vi "excel写.vi"(0 "路径":path, 1 "Table":string[][](table)=[["1", "2", "3", "4", "5", "6", "7", "8", "9", "10"], ["10", "11", "12", "13", "14", "15", "16", "17", "18", "19"], ["20", "21", "22", "23", "24", "25", "26", "27", "28", "29"], ["30", "31", "32", "33", "34", "35", "36", "37", "38", "39"]], 2 "数值":i8=1) -> ()   [LabVIEW 2011]
doc: "This VI demonstrates the use of ActiveX to write a table into a Microsoft Excel worksheet."
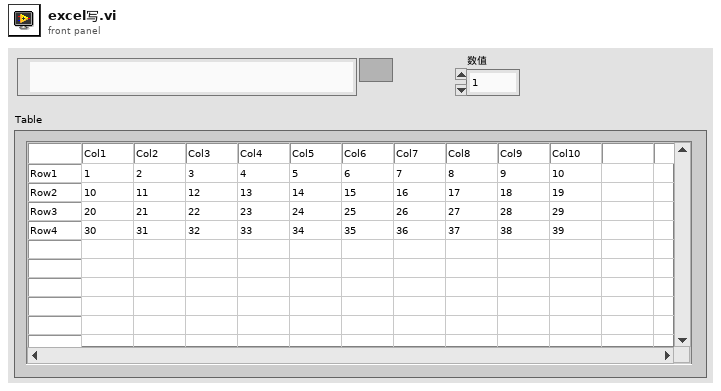
[diagram p1: front panel]
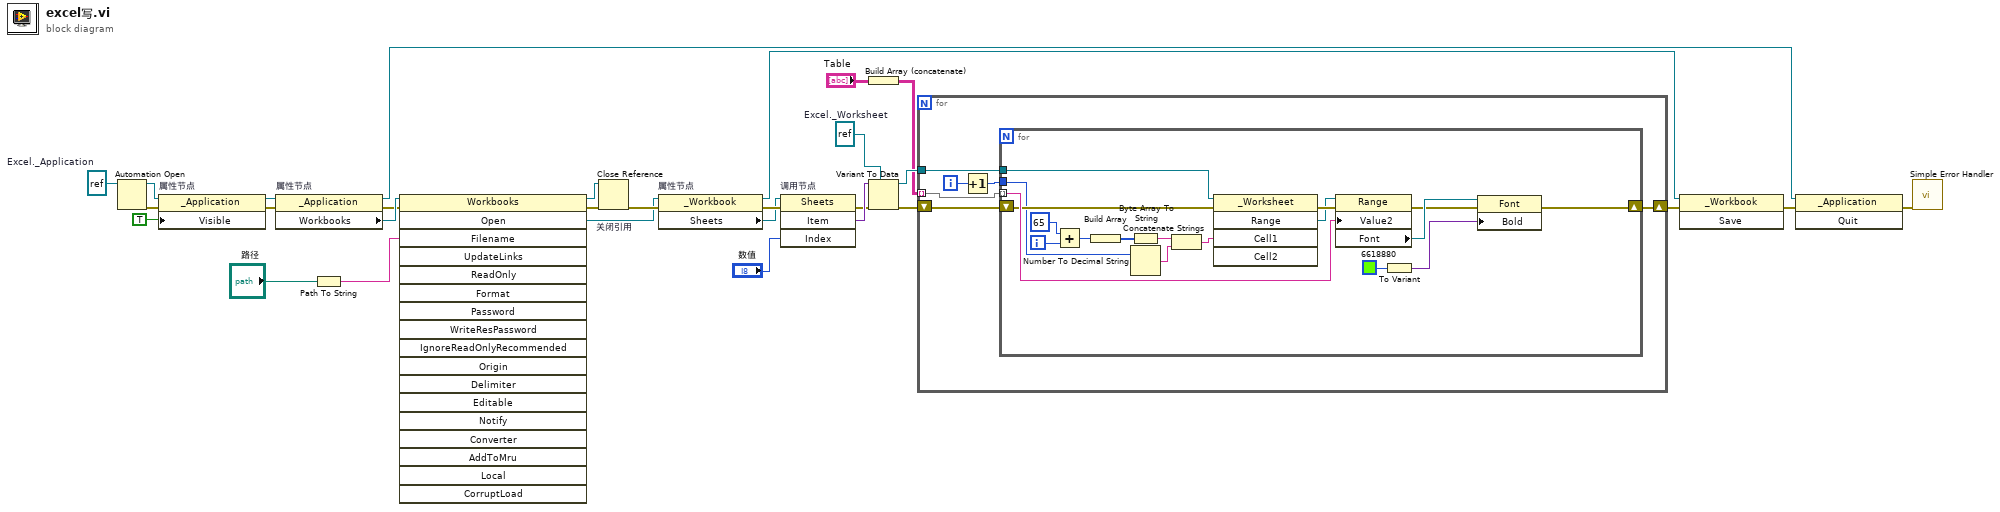
[diagram p0: block diagram]
diagram:
  w16 = refnum<k7> refnum  # Excel._Worksheet
  w27 = refnum<k7> refnum  # Excel._Application
  n1 = Automation Open(Automation Refnum=w27) -> (Automation Refnum=w28:refnum<k7>, error out=w29:errorcluster)  [unwired: 1 in, 2 out]
  n2 = property on="属性节点" class="_Application"(reference=w28, error in=w29, "Visible"=TRUE) -> (reference out=w20:refnum<k7>, error out=w22:errorcluster)
  n3 = property on="属性节点" class="_Application"(reference=w20, error in=w22) -> (reference out=w5:refnum<k7>, error out=w25:errorcluster, "Workbooks"=w26:refnum<k7>)
  n4 = Path To String(path="路径") -> (string=w9:string)
  n5 = invoke class="Workbooks" method="Open"(reference=w26, error in=w25, "Filename"=w9) -> (reference out=w23:refnum<k7>, error out=w24:errorcluster, "Open"=w18:refnum<k7>)  [unwired: 15 in, 15 out]
  n6 = Close Reference "关闭引用"(reference=w23, error in (no error)=w24) -> (error out=w19:errorcluster)
  n7 = property on="属性节点" class="_Workbook"(reference=w18, error in=w19) -> (reference out=w6:refnum<k7>, error out=w14:errorcluster, "Sheets"=w13:refnum<k7>)
  n8 = invoke on="调用节点" class="Sheets" method="Item"(reference=w13, error in=w14, "Index"="数值") -> (error out=w4:errorcluster, "Item"=w15:variant)  [unwired: 1 in, 2 out]
  n9 = Build Array (concatenate)("Table") -> (w7:string[][])
  n10 = Variant To Data(error in=w4, type=w16, Variant=w15) -> (data=w17:refnum<k7>, error out=w12:errorcluster)
  n11 = for {
    shift-right: [w34] -> w3
    shift-left: w12 -> [w35]
    tunnel: w17 -> [w33]
    tunnel: w7 -> [w30] mode=indexing
    i -> [w32]
    n12 = Increment(x=w32) -> (x+1=w31:i32)
    n13 = for {
      shift-right: [w37] -> w34
      shift-left: w35 -> [w50]
      tunnel: w33 -> [w49]
      tunnel: w31 -> [w44]
      tunnel: w30 -> [w51] mode=indexing
      i -> [w45]
      n14 = Add(x=65, y=w45) -> (x+y=w47:i32)
      n15 = Build Array(w47) -> (w46:i32[])
      n16 = Byte Array To String(unsigned byte array=w46) -> (string=w43:string)
      n17 = Number To Decimal String(number=w44) -> (decimal integer string=w42:string)  [unwired: 1 in]
      n18 = Concatenate Strings(w43, w42) -> (w41:string)
      n19 = invoke class="_Worksheet" method="Range"(reference=w49, error in=w50, "Cell1"=w41) -> (error out=w53:errorcluster, "Range"=w52:refnum<k7>)  [unwired: 2 in, 3 out]
      n20 = property class="Range"(reference=w52, error in=w53, "Value2"=w51) -> (error out=w39:errorcluster, "Font"=w40:refnum<k7>)  [unwired: 1 out]
      n21 = To Variant(anything=u32 6618880 ("颜色盒")) -> (Variant=w36:variant)
      n22 = property class="Font"(reference=w40, error in=w39, "Bold"=w36) -> (error out=w37:errorcluster)  [unwired: 1 out]
    }
  }
  n23 = invoke class="_Workbook" method="Save"(reference=w6, error in=w3) -> (error out=w2:errorcluster)  [unwired: 1 in, 2 out]
  n24 = invoke class="_Application" method="Quit"(reference=w5, error in=w2) -> (error out=w1:errorcluster)  [unwired: 1 in, 2 out]
  n25 = call <vilib>:"Simple Error Handler.vi"("error in (no error)"=w1) -> ()  [unwired: 4 in, 5 out]
